vi "teleop4.vi"() -> ()   [LabVIEW 2012]
uses:
  <vilib>/NXT/Hardware/Plugins/Tetrix DC Motor/TetrixDCMotorAddress.ctl
  <vilib>/NXT/Block Support/NXT_OutputPort.ctl
  <vilib>/NXT/NXTIO Xnodes/NXTIONodeSubVIs/LEGOStopAllMotors.vi
  <vilib>/FTC/FTC Calculate Drive Power - Arcade Left.vi
  <vilib>/NXT/NXTIO Xnodes/NXTIONodeSubVIs/LEGOMoveAllMotors.vi
  <vilib>/FTC/FTC Interpret Motor Power From Right X Axis.vi
  <vilib>/FTC/FTC Interpret Motor Power From Left X Axis.vi
  <vilib>/FTC/FTC Interpret Motor Power From Right Y Axis.vi
  <vilib>/FTC/FTC Interpret Motor Power From Left Y Axis.vi
  <vilib>/NXT/NXTIO Xnodes/NXTIONodeSubVIs/TETRIX IO Move DC Motors.vi
  <vilib>/NXT/NXTIO Xnodes/NXTIONodeSubVIs/NXTMoveMotors.vi
  <vilib>/NXT/NXTIO Xnodes/NXTIONodeSubVIs/NXTStopMotors.vi
  <vilib>/NXT/NXTIO Xnodes/NXTIONodeSubVIs/TETRIX IO Stop DC Motors.vi
  <vilib>/NXT/NXTIO Xnodes/NXTIONodeSubVIs/TETRIX IO Check Battery.vi
  <vilib>/NXT/Subs/LVHSConnector.ctl
  <vilib>/NXT/NXTIO Xnodes/NXTIOXNode/NXTIO.xnode
  <vilib>/NXT/NXTIO Xnodes/AddressXNode/NXTIOAddress.xnode
  Test.lvrbt
  <vilib>/NXT/LegoClasses/BrickReference/BrickReference.lvclass
panel:
  out "Right Multipler":i8
  out "Left Multipler":i8
  in  "Drive Power":i8=75 min=-100 max=100
  # "You may modify the code as needed for your robot. To test this program for an FTC match, open to the Remote Control Editor, select the \"Run Program\" tab, and choose \"Teleop\"."
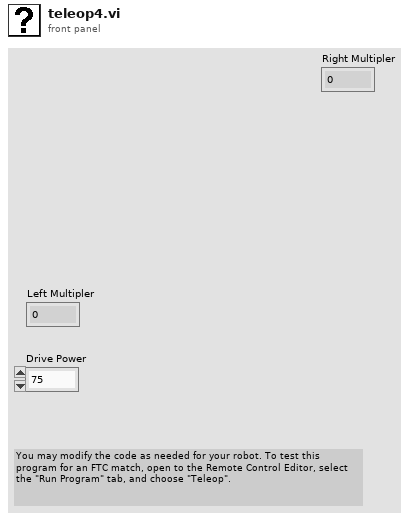
[diagram p1: front panel]
types:
  T1 = typedef "TetrixDCMotorAddress.ctl" = i32
  T2 = cluster{"TetrixDCMotor":T1, "TetrixDCMotor 2":T1}
  T3 = typedef "LVHSConnector.ctl" = refnum<class "BrickReference.lvclass">
  T4 = typedef "FTC ControllerState.ctl" = cluster{"Left X":i8, "Left Y":i8, "Right X":i8, "Right Y":i8, "Button Encoding 9-12":u8, "Button Encoding 1-8":u8, "POV":T5}
  T5 = typedef "FTC POVState.ctl" = i8
  T6 = typedef "FTC ButtonEventType.ctl" = enum16{"Pressed", "Released"}
  T7 = cluster{"Button ID":enum16{"None", "Button 1", "Button 2", "Button 3", "Button 4", "Button 5", "Button 6", "Button 7", "Button 8", "Button 9", "Button 10", "Button 11", "Button 12", "POV Up", "POV Up Right", "POV Right", "POV Down Right", "POV Down", "POV Down Left", "POV Left", "POV Up Left"}, "Event Type":T6}[]
  T8 = enum16{"None", "Button 1", "Button 2", "Button 3", "Button 4", "Button 5", "Button 6", "Button 7", "Button 8", "Button 9", "Button 10", "Button 11", "Button 12", "POV Up", "POV Up Right", "POV Right", "POV Down Right", "POV Down", "POV Down Left", "POV Left", "POV Up Left"}
  T9 = typedef "NXT_OutputPort.ctl" = u8
  T10 = typedef "FTC ButtonState.ctl" = cluster{"Button 1":bool, "Button 2":bool, "Button 3":bool, "Button 4":bool, "Button 5":bool, "Button 6":bool, "Button 7":bool, "Button 8":bool, "Button 9":bool, "Button 10":bool, "Button 11":bool, "Button 12":bool, "POV":T5}
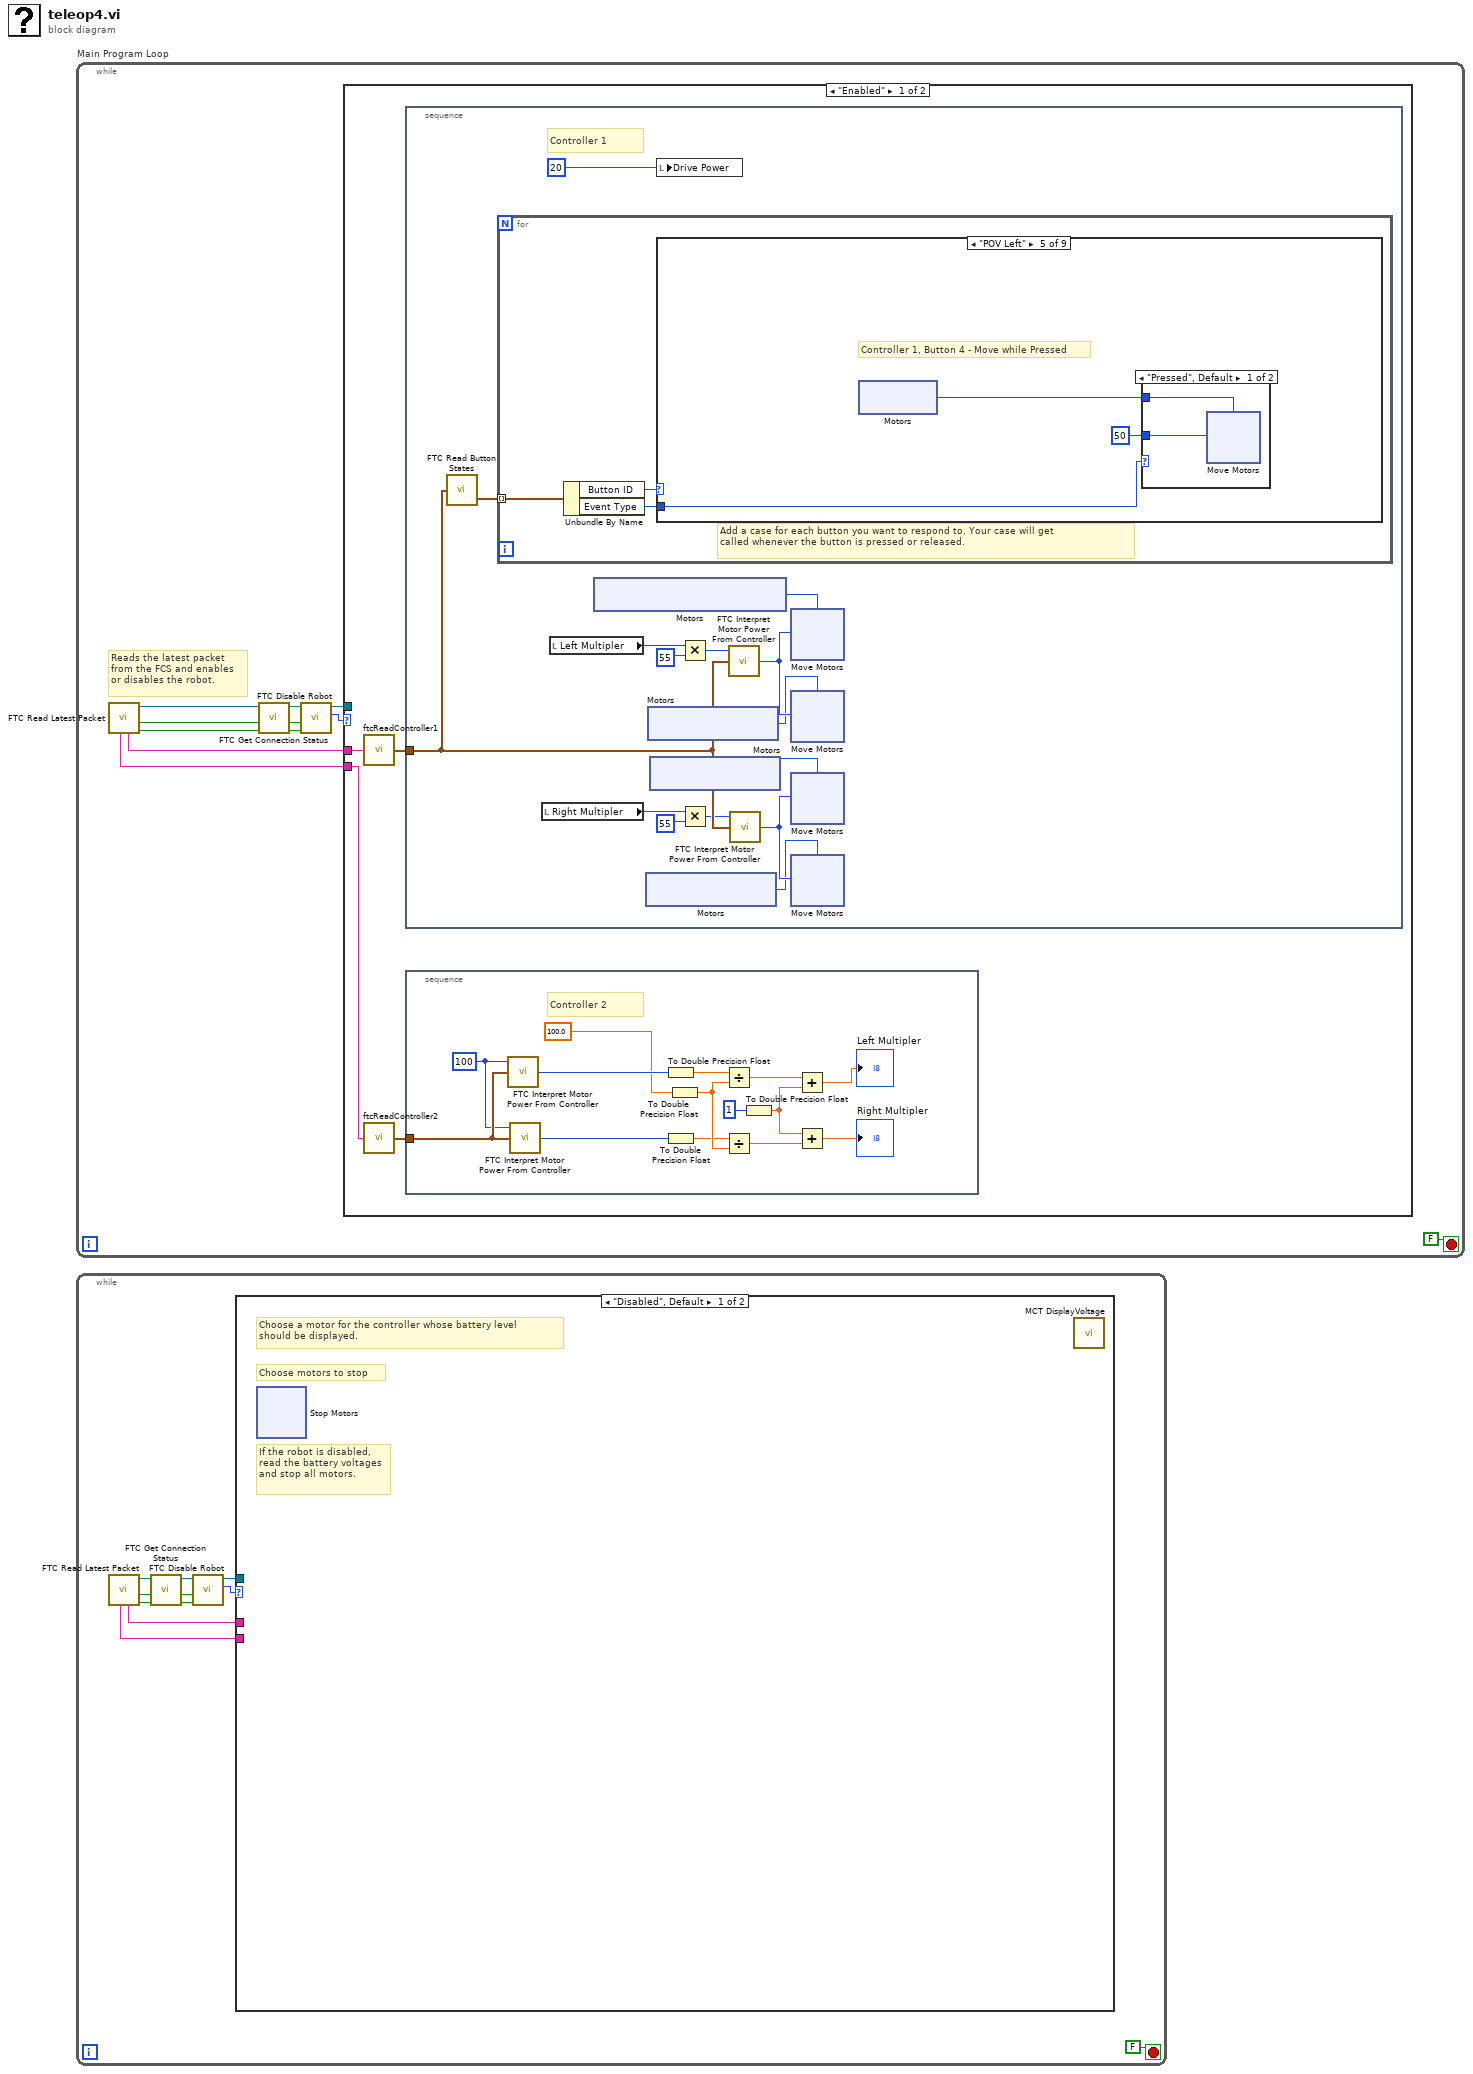
[diagram p0: block diagram]
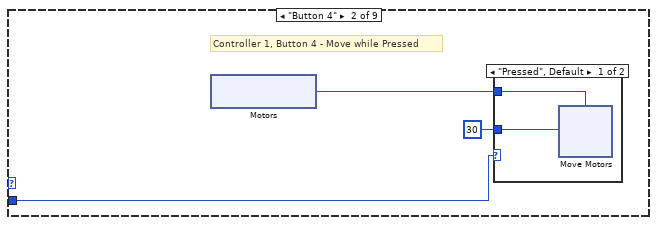
[diagram p3: hidden frame]
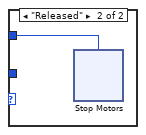
[diagram p4: hidden frame]
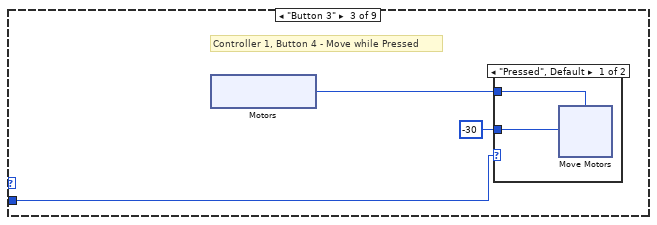
[diagram p5: hidden frame]
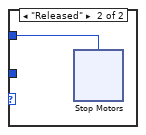
[diagram p6: hidden frame]
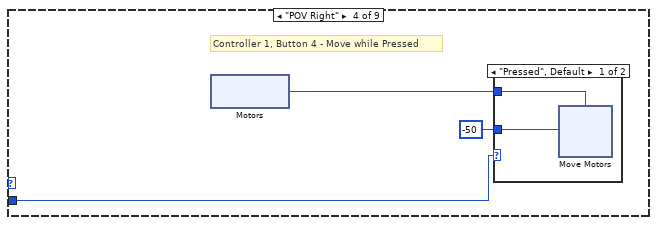
[diagram p7: hidden frame]
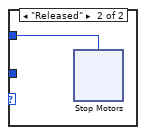
[diagram p8: hidden frame]
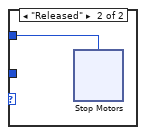
[diagram p9: hidden frame]
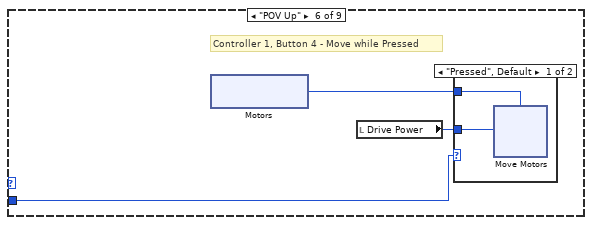
[diagram p10: hidden frame]
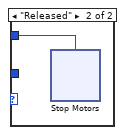
[diagram p11: hidden frame]
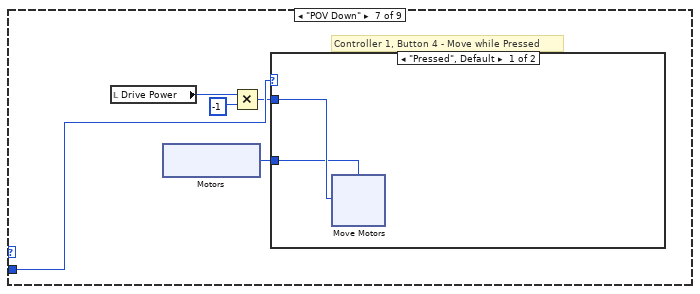
[diagram p12: hidden frame]
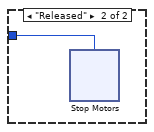
[diagram p13: hidden frame]
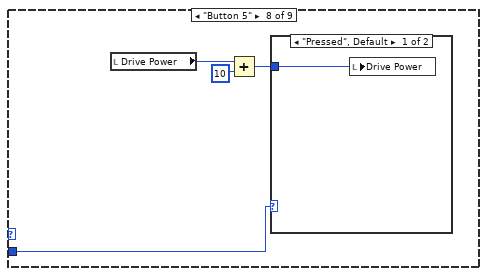
[diagram p14: hidden frame]
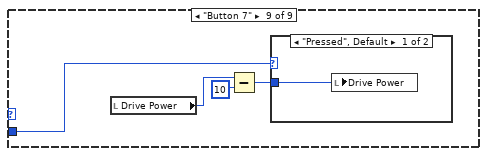
[diagram p16: hidden frame]
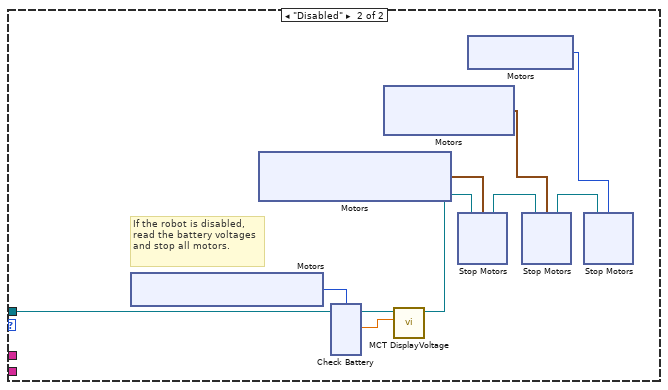
[diagram p18: hidden frame]
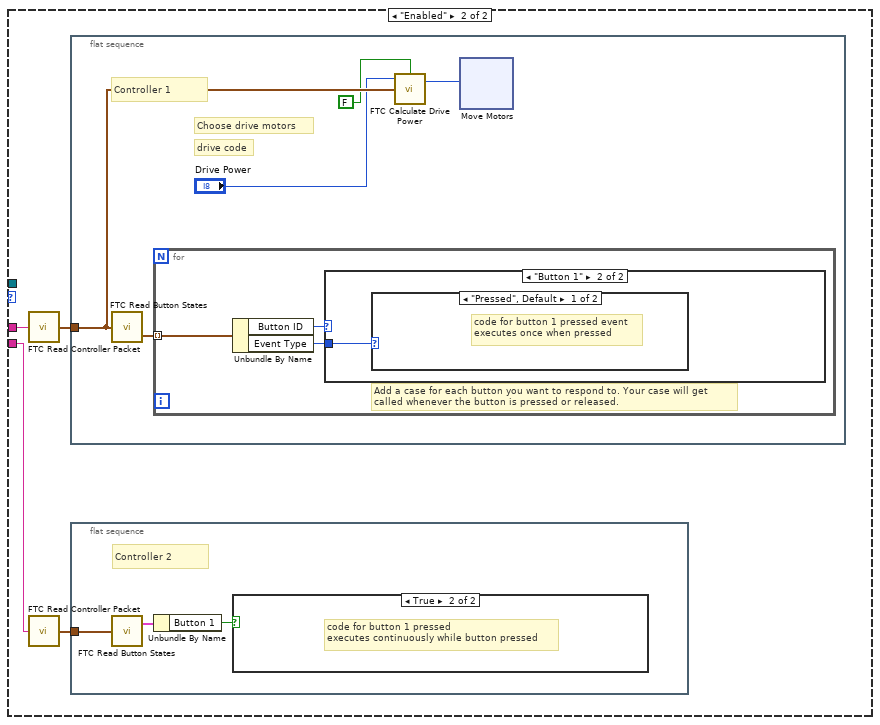
[diagram p19: hidden frame]
diagram:
  n1 = while "Main Program Loop" {
    stop <- FALSE stop-if-true
    # "Reads the latest packet\nfrom the FCS and enables\nor disables the robot."
    n2 = call <vilib>:"FTC Read Latest Packet.vi"() -> ("Packet Received?"=w8:bool, "Stopped?"=w5:bool, "NXT/EV3"=w7:T3, "Controller 1"=w10:string, "Controller 2"=w9:string)  [unwired: 6 in, 1 out]
    n3 = call <vilib>:"FTC Get Connection Status.vi"("Packet Received?"=w8, "Stopped?"=w5, "NXT/EV3"=w7) -> ("Online?"=w2:bool, "Stopped?"=w3:bool, "NXT/EV3"=w4:T3)  [unwired: 5 in]
    n4 = call <vilib>:"FTC Disable Robot.vi"("Online?"=w2, "Stopped?"=w3, "NXT/EV3"=w4) -> ("Enabled?"=w6:enum16{"Disabled", "Enabled"}, "NXT/EV3"=w1:T3)  [unwired: 3 in]
    n5 = case "disableCase" shown="\"Enabled\"" w6 {
      tunnel: w10 -> [w15 _]
      tunnel: w9 -> [w14 _]
      tunnel: w1 -> [_ w215]
      frame "Enabled" {
        n6 = call "ftcReadController1"("Packet"=w15) -> ("Controller State"=w13:T4)  [unwired: 4 in]
        n7 = call "ftcReadController2"("Packet"=w14) -> ("Controller State"=w12:T4)  [unwired: 4 in]
        n8 = stacked-sequence "controller1Actions" {
          tunnel: w13 -> [w43]
          frame #0 {
            # "Controller 1"
            n9 = call <vilib>:"FTC Read Button States.vi"("Controller State"=w43) -> ("Button Events"=w44:T7)  [unwired: 2 in, 1 out]
            n10 = for "buttonAction" {
              tunnel: w44 -> [w77] mode=indexing
              # "Add a case for each button you want to respond to. Your case will get \ncalled whenever the button is pressed or released."
              n11 = Unbundle By Name(w77) -> ("Button ID"=w79:T8, "Event Type"=w78:T6)
              n12 = case "EventCase1" shown="\"POV Left\"" w79 {
                tunnel: w78 -> [_ w82 w101 w120 w139 w158 w179 w199 w204]
                frame Default {
                  # "No Action"
                }
                frame "Button 4" {
                  # "Controller 1, Button 4 - Move while Pressed"
                  n13 = xnode "Motors"() -> ("Motor"=w80:T9)
                  n14 = case shown="\"Pressed\", Default" w82 {
                    tunnel: 30 ("Power (75)") -> [w85 _]
                    tunnel: w80 -> [w84 w93]
                    frame "Pressed", Default {
                      n15 = xnode "Move Motors"("Power/Speed 1"=w85, "Motors"=w84) -> ()  [unwired: 1 in, 1 out]
                    }
                    frame "Released" {
                      n16 = xnode "Stop Motors"("Motors"=w93) -> ()  [unwired: 1 in, 1 out]
                    }
                  }
                }
                frame "Button 3" {
                  # "Controller 1, Button 4 - Move while Pressed"
                  n17 = xnode "Motors"() -> ("Motor"=w99:T9)
                  n18 = case shown="\"Pressed\", Default" w101 {
                    tunnel: -30 ("Power (75)") -> [w104 _]
                    tunnel: w99 -> [w103 w112]
                    frame "Pressed", Default {
                      n19 = xnode "Move Motors"("Power/Speed 1"=w104, "Motors"=w103) -> ()  [unwired: 1 in, 1 out]
                    }
                    frame "Released" {
                      n20 = xnode "Stop Motors"("Motors"=w112) -> ()  [unwired: 1 in, 1 out]
                    }
                  }
                }
                frame "POV Right" {
                  # "Controller 1, Button 4 - Move while Pressed"
                  n21 = xnode "Motors"() -> ("Motor"=w118:T1)
                  n22 = case shown="\"Pressed\", Default" w120 {
                    tunnel: -50 ("Power (75)") -> [w123 _]
                    tunnel: w118 -> [w122 w131]
                    frame "Pressed", Default {
                      n23 = xnode "Move Motors"("Power/Speed 1"=w123, "Motors"=w122) -> ()  [unwired: 1 in, 1 out]
                    }
                    frame "Released" {
                      n24 = xnode "Stop Motors"("Motors"=w131) -> ()  [unwired: 1 in, 1 out]
                    }
                  }
                }
                frame "POV Left" {
                  # "Controller 1, Button 4 - Move while Pressed"
                  n25 = xnode "Motors"() -> ("Motor"=w137:T1)
                  n26 = case shown="\"Pressed\", Default" w139 {
                    tunnel: 50 ("Power (75)") -> [w142 _]
                    tunnel: w137 -> [w141 w150]
                    frame "Pressed", Default {
                      n27 = xnode "Move Motors"("Power/Speed 1"=w142, "Motors"=w141) -> ()  [unwired: 1 in, 1 out]
                    }
                    frame "Released" {
                      n28 = xnode "Stop Motors"("Motors"=w150) -> ()  [unwired: 1 in, 1 out]
                    }
                  }
                }
                frame "POV Up" {
                  # "Controller 1, Button 4 - Move while Pressed"
                  n29 = xnode "Motors"() -> ("Motor"=w157:T1)
                  n30 = local read "Drive Power"() -> (w156:i8)
                  n31 = case shown="\"Pressed\", Default" w158 {
                    tunnel: w156 -> [w161 _]
                    tunnel: w157 -> [w160 w169]
                    frame "Pressed", Default {
                      n32 = xnode "Move Motors"("Power/Speed 1"=w161, "Motors"=w160) -> ()  [unwired: 1 in, 1 out]
                    }
                    frame "Released" {
                      n33 = xnode "Stop Motors"("Motors"=w169) -> ()  [unwired: 1 in, 1 out]
                    }
                  }
                }
                frame "POV Down" {
                  # "Controller 1, Button 4 - Move while Pressed"
                  n34 = local read "Drive Power"() -> (w176:i8)
                  n35 = xnode "Motors"() -> ("Motor"=w178:T1)
                  n36 = Multiply(x=w176, y=-1) -> (x*y=w175:i32)
                  n37 = case shown="\"Pressed\", Default" w179 {
                    tunnel: w175 -> [w182 _]
                    tunnel: w178 -> [w181 w190]
                    frame "Pressed", Default {
                      n38 = xnode "Move Motors"("Power/Speed 1"=w182, "Motors"=w181) -> ()  [unwired: 1 in, 1 out]
                    }
                    frame "Released" {
                      n39 = xnode "Stop Motors"("Motors"=w190) -> ()  [unwired: 1 in, 1 out]
                    }
                  }
                }
                frame "Button 5" {
                  n40 = local read "Drive Power"() -> (w198:i8)
                  n41 = Add(x=w198, y=10) -> (x+y=w196:i32)
                  n42 = case shown="\"Pressed\", Default" w199 {
                    tunnel: w196 -> [w200 _]
                    frame "Pressed", Default {
                      n43 = local write "Drive Power"(w200) -> ()
                    }
                    frame "Released" {
                    }
                  }
                }
                frame "Button 7" {
                  n44 = local read "Drive Power"() -> (w202:i8)
                  n45 = Subtract(x=w202, y=10) -> (x-y=w201:i32)
                  n46 = case shown="\"Pressed\", Default" w204 {
                    tunnel: w201 -> [w205 _]
                    frame "Pressed", Default {
                      n47 = local write "Drive Power"(w205) -> ()
                    }
                    frame "Released" {
                    }
                  }
                }
              }
            }
            n48 = local read "Right Multipler"() -> (w35:i8)
            n49 = local read "Left Multipler"() -> (w30:i8)
            n50 = xnode "Motors"() -> ("Motor"=w42:T1)
            n51 = xnode "Motors"() -> ("Motor"=w38:T1)
            n52 = xnode "Motors"() -> ("Motor"=w39:T1)
            n53 = xnode ("Motors")() -> ("Motor"=w37:T1)
            n54 = local write "Drive Power"(i8 20 ("Drive Power")) -> ()
            n55 = Multiply(x=w30, y=i8 55 ("Power Level (50)")) -> (x*y=w31:i8)
            n56 = Multiply(x=w35, y=i8 55 ("Power Level (50)")) -> (x*y=w33:i8)
            n57 = call-poly <vilib>:"FTC Interpret Motor Power From Controller.vi"("Controller State"=w43, "Power Level (50)"=w31) -> ("Power"=w41:i8)  [unwired: 1 in]
            n58 = call-poly <vilib>:"FTC Interpret Motor Power From Controller.vi"("Controller State"=w43, "Power Level (50)"=w33) -> ("Power"=w40:i8)  [unwired: 1 in]
            n59 = xnode "Move Motors"("Power/Speed 1"=w41, "Motors"=w42) -> ()  [unwired: 1 in, 1 out]
            n60 = xnode "Move Motors"("Power/Speed 1"=w41, "Motors"=w39) -> ()  [unwired: 1 in, 1 out]
            n61 = xnode ("Move Motors")("Power/Speed 1"=w40, "Motors"=w37) -> ()  [unwired: 1 in, 1 out]
            n62 = xnode "Move Motors"("Power/Speed 1"=w40, "Motors"=w38) -> ()  [unwired: 1 in, 1 out]
          }
        }
        n63 = stacked-sequence "controller2Actions" {
          tunnel: w12 -> [w29]
          frame #0 {
            w28 = i8 100 ("Power Level (50)")
            # "Controller 2"
            n64 = call-poly <vilib>:"FTC Interpret Motor Power From Controller.vi"("Controller State"=w29, "Power Level (50)"=w28) -> ("Power"=w24:i8)  [unwired: 1 in]
            n65 = call-poly <vilib>:"FTC Interpret Motor Power From Controller.vi"("Controller State"=w29, "Power Level (50)"=w28) -> ("Power"=w25:i8)  [unwired: 1 in]
            n66 = To Double Precision Float(number=w24) -> (double precision float=w18:dbl)
            n67 = To Double Precision Float(number=w25) -> (double precision float=w16:dbl)
            n68 = To Double Precision Float(number=100.0) -> (double precision float=w17:dbl)
            n69 = Divide(x=w18, y=w17) -> (x/y=w20:dbl)
            n70 = Divide(x=w16, y=w17) -> (x/y=w21:dbl)
            n71 = To Double Precision Float(number=i8 1 ("y")) -> (double precision float=w22:dbl)
            n72 = Add(x=w20, y=w22) -> (x+y=→"Left Multipler":dbl)
            n73 = Add(x=w22, y=w21) -> (x+y=→"Right Multipler":dbl)
          }
        }
      }
      frame "Disabled" {
        # "If the robot is disabled, read the battery voltages and stop all motors."
        n74 = xnode ("Motors")() -> ("Motor"=w214:T1)
        n75 = xnode "Motors"() -> ("Motor"=w211:cluster{"TetrixDCMotor":T1, "TetrixDCMotor":T1})
        n76 = xnode ("Check Battery")("Motors"=w214, "NXT/EV3"=w215) -> ("Voltage 1"=w213:sgl, "NXT/EV3"=w212:T3)
        n77 = xnode "Motors"() -> ("Motor"=w209:cluster{"TetrixDCMotor":T1, "TetrixDCMotor":T1})
        n78 = call <vilib>:"MCT DisplayVoltage.vi"("Motor Voltage"=w213, "NXT/EV3"=w212) -> ("NXT/EV3"=w210:T3)  [unwired: 9 in]
        n79 = xnode "Stop Motors"("Motors"=w211, "NXT/EV3"=w210) -> ("NXT/EV3"=w208:T3)
        n80 = xnode "Motors"() -> ("Motor"=w207:T9)
        n81 = xnode "Stop Motors"("Motors"=w209, "NXT/EV3"=w208) -> ("NXT/EV3"=w206:T3)
        n82 = xnode "Stop Motors"("Motors"=w207, "NXT/EV3"=w206) -> ()  [unwired: 1 out]
      }
    }
  }
  n83 = while {
    stop <- FALSE stop-if-true
    n84 = call <vilib>:"FTC Read Latest Packet.vi"() -> ("Packet Received?"=w250:bool, "Stopped?"=w249:bool, "NXT/EV3"=w248:T3, "Controller 1"=w242:string, "Controller 2"=w241:string)  [unwired: 6 in, 1 out]
    n85 = call <vilib>:"FTC Get Connection Status.vi"("Packet Received?"=w250, "Stopped?"=w249, "NXT/EV3"=w248) -> ("Online?"=w247:bool, "Stopped?"=w246:bool, "NXT/EV3"=w245:T3)  [unwired: 5 in]
    n86 = call <vilib>:"FTC Disable Robot.vi"("Online?"=w247, "Stopped?"=w246, "NXT/EV3"=w245) -> ("Enabled?"=w244:enum16{"Disabled", "Enabled"}, "NXT/EV3"=w243:T3)  [unwired: 3 in]
    n87 = case shown="\"Disabled\", Default" w244 {
      tunnel: w243 -> [_ _]
      tunnel: w242 -> [_ w259]
      tunnel: w241 -> [_ w258]
      frame "Disabled", Default {
        # "Choose motors to stop"
        # "Choose a motor for the controller whose battery level \nshould be displayed."
        # "If the robot is disabled, read the battery voltages and stop all motors."
        n88 = xnode "Stop Motors"() -> ()  [unwired: 2 in, 1 out]
        n89 = call <vilib>:"MCT DisplayVoltage.vi"() -> ()  [unwired: 11 in, 1 out]
      }
      frame "Enabled" {
        n90 = call <vilib>:"FTC Read Controller Packet.vi"("Packet"=w259) -> ("Controller State"=w256:T4)  [unwired: 4 in]
        n91 = call <vilib>:"FTC Read Controller Packet.vi"("Packet"=w258) -> ("Controller State"=w257:T4)  [unwired: 4 in]
        n92 = flat-sequence {
          tunnel: w256 -> [w266]
          frame #0 {
            # "Choose drive motors"
            # "drive code"
            # "Controller 1"
            n93 = call <vilib>:"FTC Read Button States.vi"("Controller State"=w266) -> ("Button Events"=w267:T7)  [unwired: 2 in, 1 out]
            n94 = for {
              tunnel: w267 -> [w277] mode=indexing
              # "Add a case for each button you want to respond to. Your case will get \ncalled whenever the button is pressed or released."
              n95 = Unbundle By Name(w277) -> ("Button ID"=w276:T8, "Event Type"=w275:T6)
              n96 = case shown="\"Button 1\"" w276 {
                tunnel: w275 -> [_ w278]
                frame "None", Default {
                }
                frame "Button 1" {
                  n97 = case shown="\"Pressed\", Default" w278 {
                    frame "Pressed", Default {
                      # "code for button 1 pressed event\nexecutes once when pressed"
                    }
                    frame "Released" {
                    }
                  }
                }
              }
            }
            n98 = call-poly <vilib>:"FTC Calculate Drive Power.vi"("Reverse"=FALSE, "Controller State"=w266, "Power Level (50)"="Drive Power") -> ("Left Motor Power"=w263:i8)  [unwired: 1 in, 1 out]
            n99 = xnode "Move Motors"("Power/Speed 1"=w263) -> ()  [unwired: 2 in, 1 out]
          }
        }
        n100 = flat-sequence {
          tunnel: w257 -> [w262]
          frame #0 {
            # "Controller 2"
            n101 = call <vilib>:"FTC Read Button States.vi"("Controller State"=w262) -> ("Button States"=w261:T10)  [unwired: 2 in, 1 out]
            n102 = Unbundle By Name(w261) -> ("Button 1"=w260:bool)
            n103 = case shown="True" w260 {
              frame False {
              }
              frame True {
                # "code for button 1 pressed\nexecutes continuously while button pressed"
              }
            }
          }
        }
      }
    }
  }
